vi "Update Main State.vi"(8 "error in":errorcluster, 10 "Loading":bool, 11 "Manual UI in":refnum<class "Manual UI.lvclass">) -> (0 "error out":errorcluster, 3 "Manual UI out":refnum<class "Manual UI.lvclass">)   [LabVIEW 2023, in "Manual UI.lvlib" / "Manual UI.lvclass"]
uses:
  Project/Manual UI.lvclass
  builds/Engine/Engine.lvlibp/Custom Controls/System Status.ctl
  builds/Engine/Engine.lvlibp/Project/Engine.lvclass
  C:/Users/Public/Documents/Development/builds/Engine/Engine.lvlibp/Project/Engine.lvclass
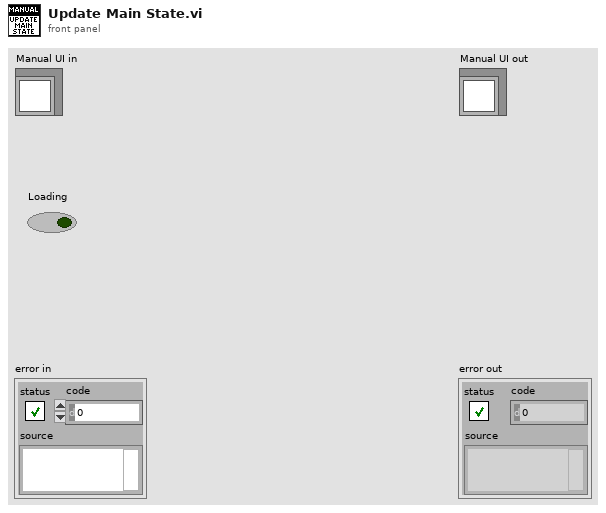
[diagram p1: front panel]
types:
  T1 = typedef "Engine.lvlibp/Engine.lvclass/System Status.ctl" = enum16{"Logged Off", "UUT_Info_Missing", "Idle", "Error", "Warning", "Loading", "Config", "Manual", "Automation", "Report_View", "Previous"}
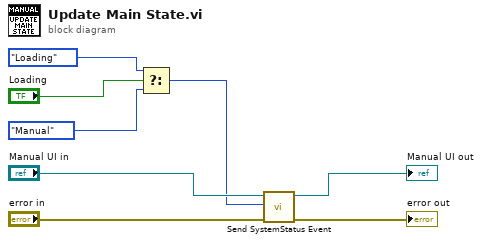
[diagram p0: block diagram]
diagram:
  n1 = Select(t=System_Status."Loading" ("SystemStatus"), s="Loading", f=System_Status."Manual" ("SystemStatus")) -> (s? t:f=w1:T1)
  n2 = call "Send SystemStatus Event.vi"("error in"="error in", "SystemStatus"=w1, "Engine in"="Manual UI in") -> ("error out"=→"error out":errorcluster, "Engine out"=→"Manual UI out":refnum<class "Manual UI.lvclass">)  [unwired: 7 in]
